vi "death.vi"(10 "Game Parameters":T1, 11 "Arrays and Heights":T2={"Score Array"=[], "Lowest high score"=0.0, "Score"=0.0, "Ceiling"=0.0, "Floor"=0.0, "Ceiling Array"=[], "Floor array"=[], "Helicopter height"=0.0, "Helicopter array"=[], "Fuel"=0.0, "Fuel array"=[], "fuel counter"=0, "obstacle counter"=0, "Obstacle array"=[], "helicopter v_0"=0.0, "helicopter a_0"=0.0, "Obstacle height"=300.0}) -> (3 "Death?":bool)   [LabVIEW 2017]
uses:
  controls/arrays and heights.ctl
  controls/scores.ctl
  controls/game parameters.ctl
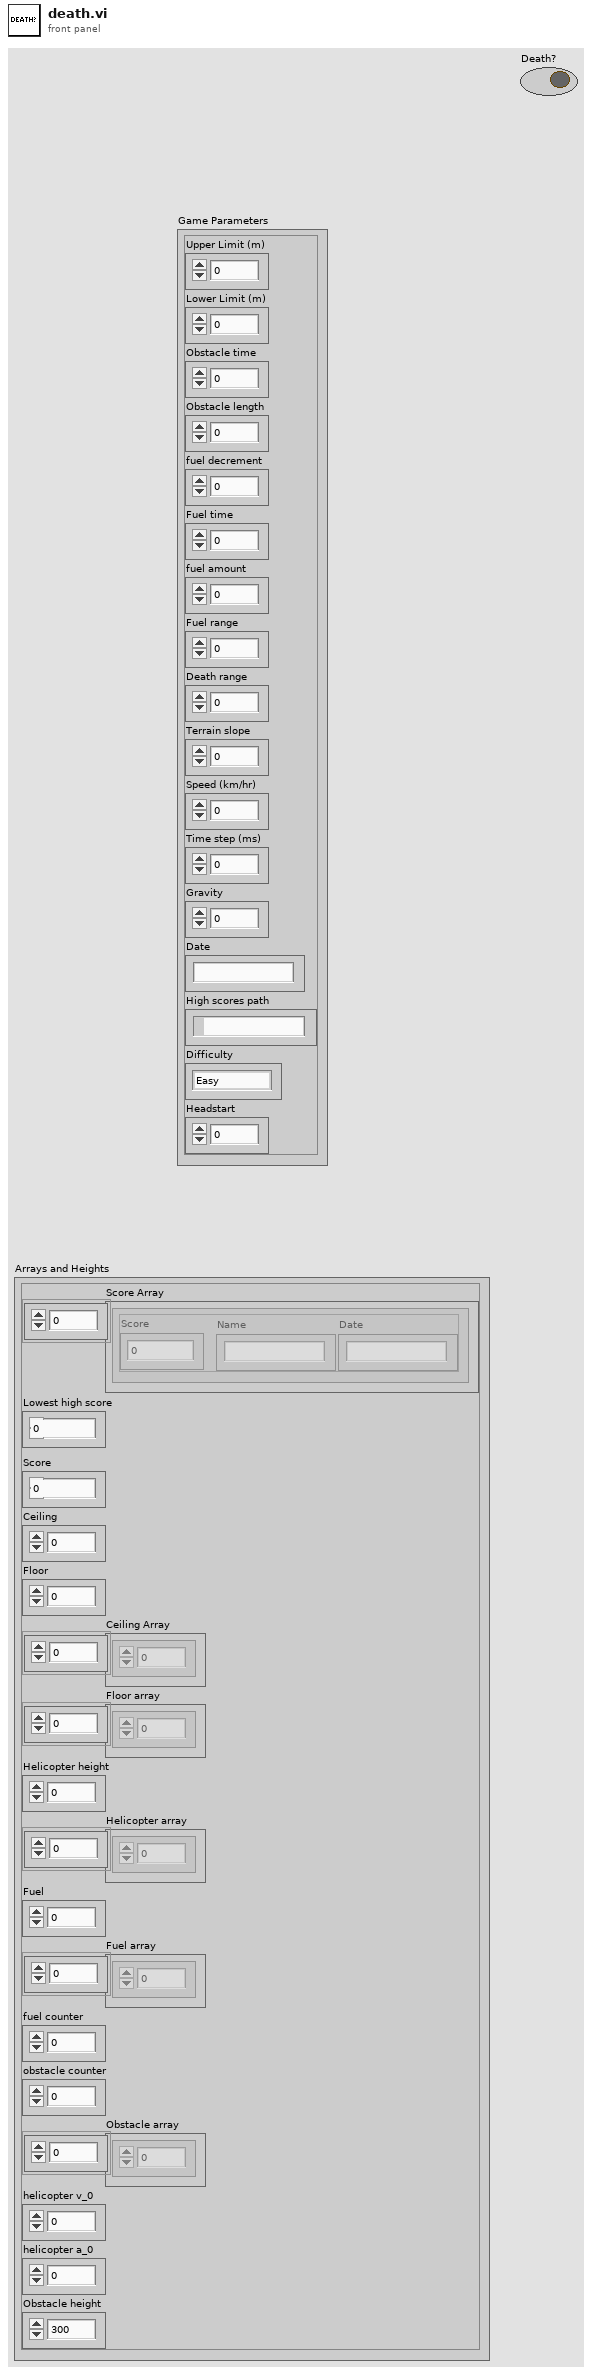
[diagram p1: front panel]
types:
  T1 = typedef "game parameters.ctl" = cluster{"Upper Limit (m)":dbl, "Lower Limit (m)":dbl, "Obstacle time":dbl, "Obstacle length":dbl, "fuel decrement":dbl, "Fuel time":dbl, "fuel amount":dbl, "Fuel range":i32, "Death range":i32, "Terrain slope":dbl, "Speed (km/hr)":dbl, "Time step (ms)":u32, "Gravity":dbl, "Date":string, "High scores path":path, "Difficulty":enum16{"Easy", "Normal", "Hard"}, "Headstart":u32}
  T2 = typedef "arrays and heights.ctl" = cluster{"Score Array":T3[], "Lowest high score":dbl, "Score":dbl, "Ceiling":dbl, "Floor":dbl, "Ceiling Array":dbl[], "Floor array":dbl[], "Helicopter height":dbl, "Helicopter array":dbl[], "Fuel":dbl, "Fuel array":dbl[], "fuel counter":i32, "obstacle counter":i32, "Obstacle array":dbl[], "helicopter v_0":dbl, "helicopter a_0":dbl, "Obstacle height":dbl}
  T3 = typedef "scores.ctl" = cluster{"Score":dbl, "Name":string, "Date":string}
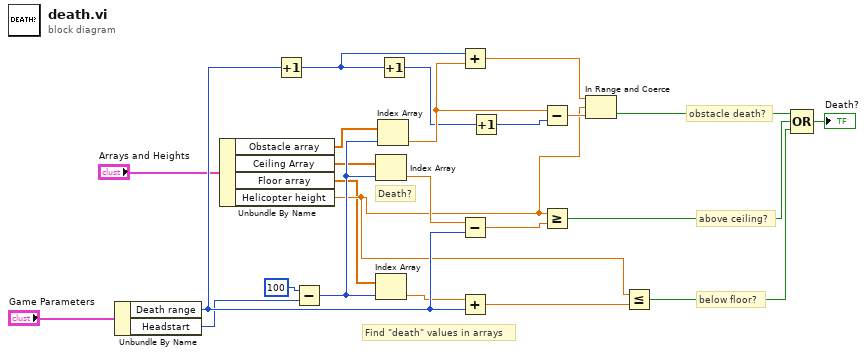
[diagram p0: block diagram]
diagram:
  # "Death?"
  # "obstacle death?"
  # "Find \"death\" values in arrays"
  # "below floor?"
  # "above ceiling?"
  n1 = Unbundle By Name("Game Parameters") -> ("Death range"=w21:i32, "Headstart"=w20:u32)
  n2 = Unbundle By Name("Arrays and Heights") -> ("Obstacle array"=w23:dbl[], "Ceiling Array"=w2:dbl[], "Floor array"=w1:dbl[], "Helicopter height"=w4:dbl)
  n3 = Increment(x=w21) -> (x+1=w18:i32)
  n4 = Subtract(x=u32 100, y=w20) -> (x-y=w19:u32)
  n5 = Index Array(array=w2, index=w19) -> (element=w6:dbl)
  n6 = Index Array(array=w1, index=w19) -> (element=w5:dbl)
  n7 = Index Array(array=w23, index=w19) -> (element=w17:dbl)
  n8 = Increment(x=w18) -> (x+1=w11:i32)
  n9 = Add(x=w18, y=w17) -> (x+y=w12:dbl)
  n10 = Subtract(x=w6, y=w21) -> (x-y=w10:dbl)
  n11 = Add(x=w5, y=w21) -> (x+y=w9:dbl)
  n12 = Increment(x=w11) -> (x+1=w13:i32)
  n13 = Subtract(x=w17, y=w13) -> (x-y=w8:dbl)
  n14 = Greater Or Equal?(x=w4, y=w10) -> (x >= y?=w15:bool)
  n15 = In Range and Coerce(upper limit=w12, x=w4, lower limit=w8) -> (In Range?=w16:bool)  [unwired: 1 out]
  n16 = Less Or Equal?(x=w4, y=w9) -> (x <= y?=w14:bool)
  n17 = Compound Arithmetic op=OR(w16, w15, w14) -> (→"Death?":bool)
